vi "Word_Quit.vi"(0 "Word._Application in":refnum<k7>, 5 "Word._Document in":refnum<k7>, 7 "save changes?":bool, 9 "wait until print completed?":bool, 11 "error in(no error)":errorcluster, 12 "Close Application":bool, 13 "Close Report":bool) -> (4 "Word._Application out":refnum<k7>, 6 "Word._Document out":refnum<k7>, 15 "error out":errorcluster)   [LabVIEW 2010, in "NI_ReportGenerationToolkit.lvlib"]
uses:
  <vilib>/addons/_office/NI_ReportGenerationToolkit.lvlib
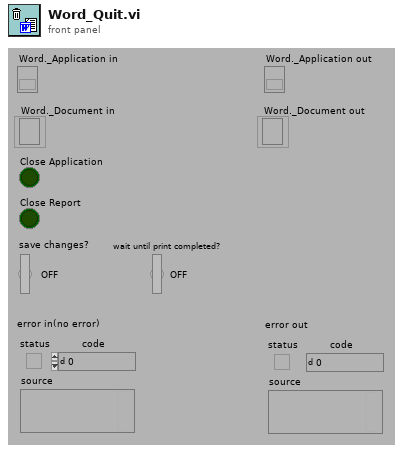
[diagram p1: front panel]
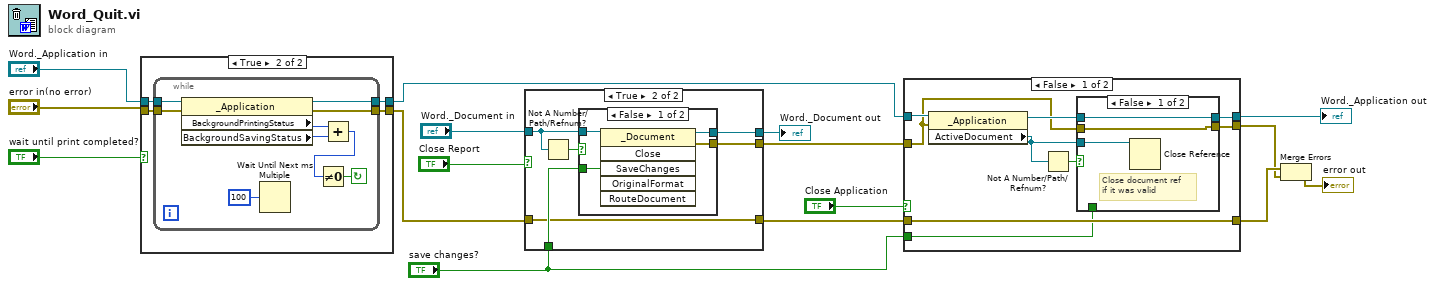
[diagram p0: block diagram]
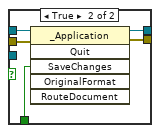
[diagram p4: hidden frame]
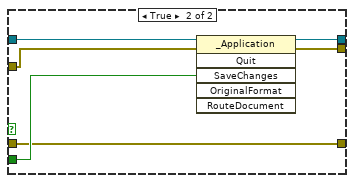
[diagram p5: hidden frame]
diagram:
  n1 = case shown="True" "wait until print completed?" {
    tunnel: [w17 w22] -> w8
    tunnel: "error in(no error)" -> [w17 w21]
    tunnel: "Word._Application in" -> [w18 w20]
    tunnel: [w18 w19] -> w10
    frame False {
    }
    frame True {
      n2 = while {
        tunnel: [w28] -> w19
        tunnel: w20 -> [w29]
        tunnel: w21 -> [w30]
        tunnel: [w31] -> w22
        stop <- w27 continue-if-true
        n3 = property class="_Application"(reference=w29, error in=w30) -> (reference out=w28:refnum<k7>, error out=w31:errorcluster, "BackgroundPrintingStatus"=w24:i32, "BackgroundSavingStatus"=w25:i32)
        n4 = Wait Until Next ms Multiple(millisecond multiple=u32 100) -> ()  [unwired: 1 out]
        n5 = Add(x=w24, y=w25) -> (x+y=w23:i32)
        n6 = Not Equal To 0?(x=w23) -> (x != 0?=w27:bool)
      }
    }
  }
  n7 = case shown="True" "Close Report" {
    tunnel: "Word._Document in" -> [w33 w35]
    tunnel: [w33 w39] -> w9
    tunnel: w8 -> [w32 w37]
    tunnel: "save changes?" -> [_ w38]
    tunnel: [w32 w37] -> w5
    tunnel: [_ w36] -> w3
    frame False {
    }
    frame True {
      n8 = Not A Number/Path/Refnum?(number/path/refnum=w35) -> (NaN/Path/Refnum?=w34:bool)
      n9 = case shown="False" w34 {
        tunnel: w35 -> [w43 w44]
        tunnel: [w42 w44] -> w39
        tunnel: w38 -> [w41 _]
        tunnel: [w40 _] -> w36
        frame False {
          n10 = invoke class="_Document" method="Close"(reference=w43, "SaveChanges"=w41) -> (reference out=w42:refnum<k7>, error out=w40:errorcluster)  [unwired: 4 in, 4 out]
        }
        frame True {
        }
      }
    }
  }
  "Word._Document out" <- w9
  n11 = case shown="False" "Close Application" {
    tunnel: [w52 w65] -> w1
    tunnel: [w51 w67] -> w16
    tunnel: w10 -> [w49 w66]
    tunnel: w5 -> [w53 w63]
    tunnel: "save changes?" -> [w50 w64]
    tunnel: [w53 w63] -> w2
    tunnel: w3 -> [w46 w62]
    frame False {
      n12 = property class="_Application"(reference=w49, error in=w46) -> (reference out=w48:refnum<k7>, "ActiveDocument"=w45:refnum<k7>)  [unwired: 1 out]
      n13 = Not A Number/Path/Refnum?(number/path/refnum=w45) -> (NaN/Path/Refnum?=w47:bool)
      n14 = case shown="False" w47 {
        tunnel: [w55 w61] -> w52
        tunnel: [w56 w60] -> w51
        tunnel: w48 -> [w56 w59]
        tunnel: w50 -> [_ w58]
        tunnel: w46 -> [w55 w57]
        tunnel: w45 -> [w54 _]
        frame False {
          # "Close document ref\nif it was valid"
          n15 = Close Reference(reference=w54) -> ()  [unwired: 1 in, 1 out]
        }
        frame True {
          n16 = invoke class="_Application" method="Quit"(reference=w59, error in=w57, "SaveChanges"=w58) -> (reference out=w60:refnum<k7>, error out=w61:errorcluster)  [unwired: 3 in, 4 out]
        }
      }
    }
    frame True {
      n17 = invoke class="_Application" method="Quit"(reference=w66, error in=w62, "SaveChanges"=w64) -> (reference out=w67:refnum<k7>, error out=w65:errorcluster)  [unwired: 3 in, 4 out]
    }
  }
  "Word._Application out" <- w16
  n18 = Merge Errors(w2, w1) -> (→"error out":errorcluster)
